vi "Material-ConfigPage-Shutdown.vi"(0 "Configuration Page":refnum<class "Material-ConfigPage.lvclass">, 11 "error in":errorcluster) -> (15 "error out":errorcluster)   [LabVIEW 2013, in "Material-ConfigPage.lvclass"]
uses:
  Material-ConfigPage.lvclass
  Material-ConfigPage.lvclass/Material-ConfigPage.ctl
  Reuse Library/featherweight/Core/Messaging/Messenger.Actor/FTW-Messenger-Actor.lvclass
panel:
  # "Inputs"
  # "Outputs"
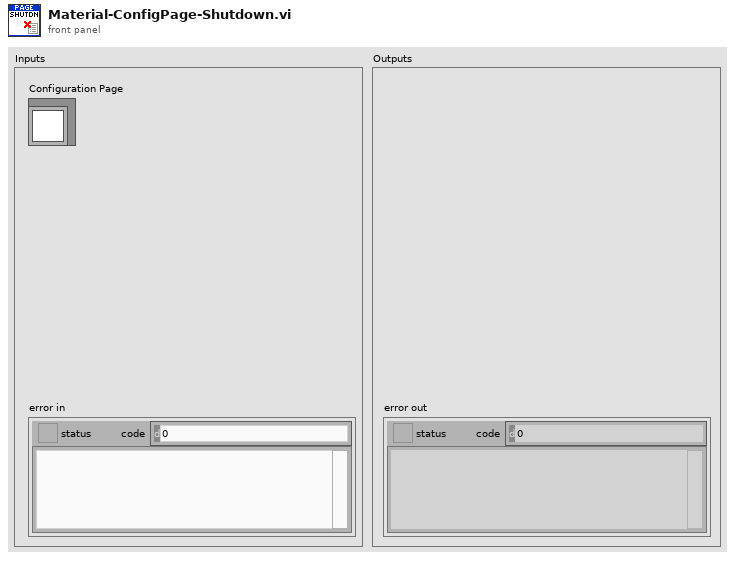
[diagram p1: front panel]
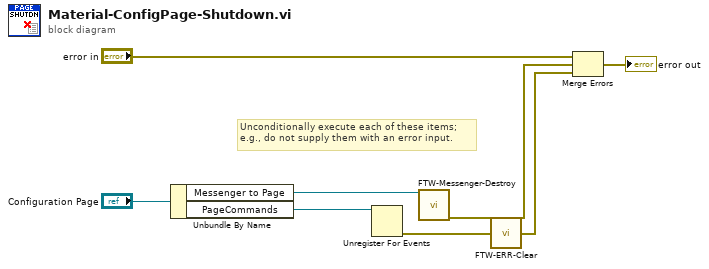
[diagram p0: block diagram]
diagram:
  # "Unconditionally execute each of these items;\ne.g., do not supply them with an error input."
  n1 = Unbundle By Name("Configuration Page") -> ("Messenger to Page"=w6:refnum<class "FTW-Messenger-Actor.lvclass">, "PageCommands"=w1:refnum<event-registration>)
  n2 = Unregister For Events(event registration refnum=w1) -> (error out=w3:errorcluster)  [unwired: 1 in]
  n3 = call-dynamic "FTW-Messenger-Destroy.vi"("Messenger"=w6) -> ("error out"=w5:errorcluster)  [unwired: 14 in]
  n4 = call "FTW-ERR-Clear.vi"("error to snuff"=w3) -> ("no error"=w2:errorcluster)
  n5 = Merge Errors("error in", w5, w2) -> (→"error out":errorcluster)
